vi "Data Logger.vi"(10 "logging rate (ms)":u32, 11 "YOU WANT TO LOG?":bool) -> ()   [LabVIEW 2016]
uses:
  Globale Variablen VI/AutonomousMode.vi
  Globale Variablen VI/Logging Globale Variable.vi
  Globale Variablen VI/Global Variables.vi
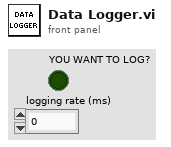
[diagram p1: front panel]
types:
  T1 = enum16{"open", "replace", "create", "open or create", "replace or create", "replace or create with confirmation"}
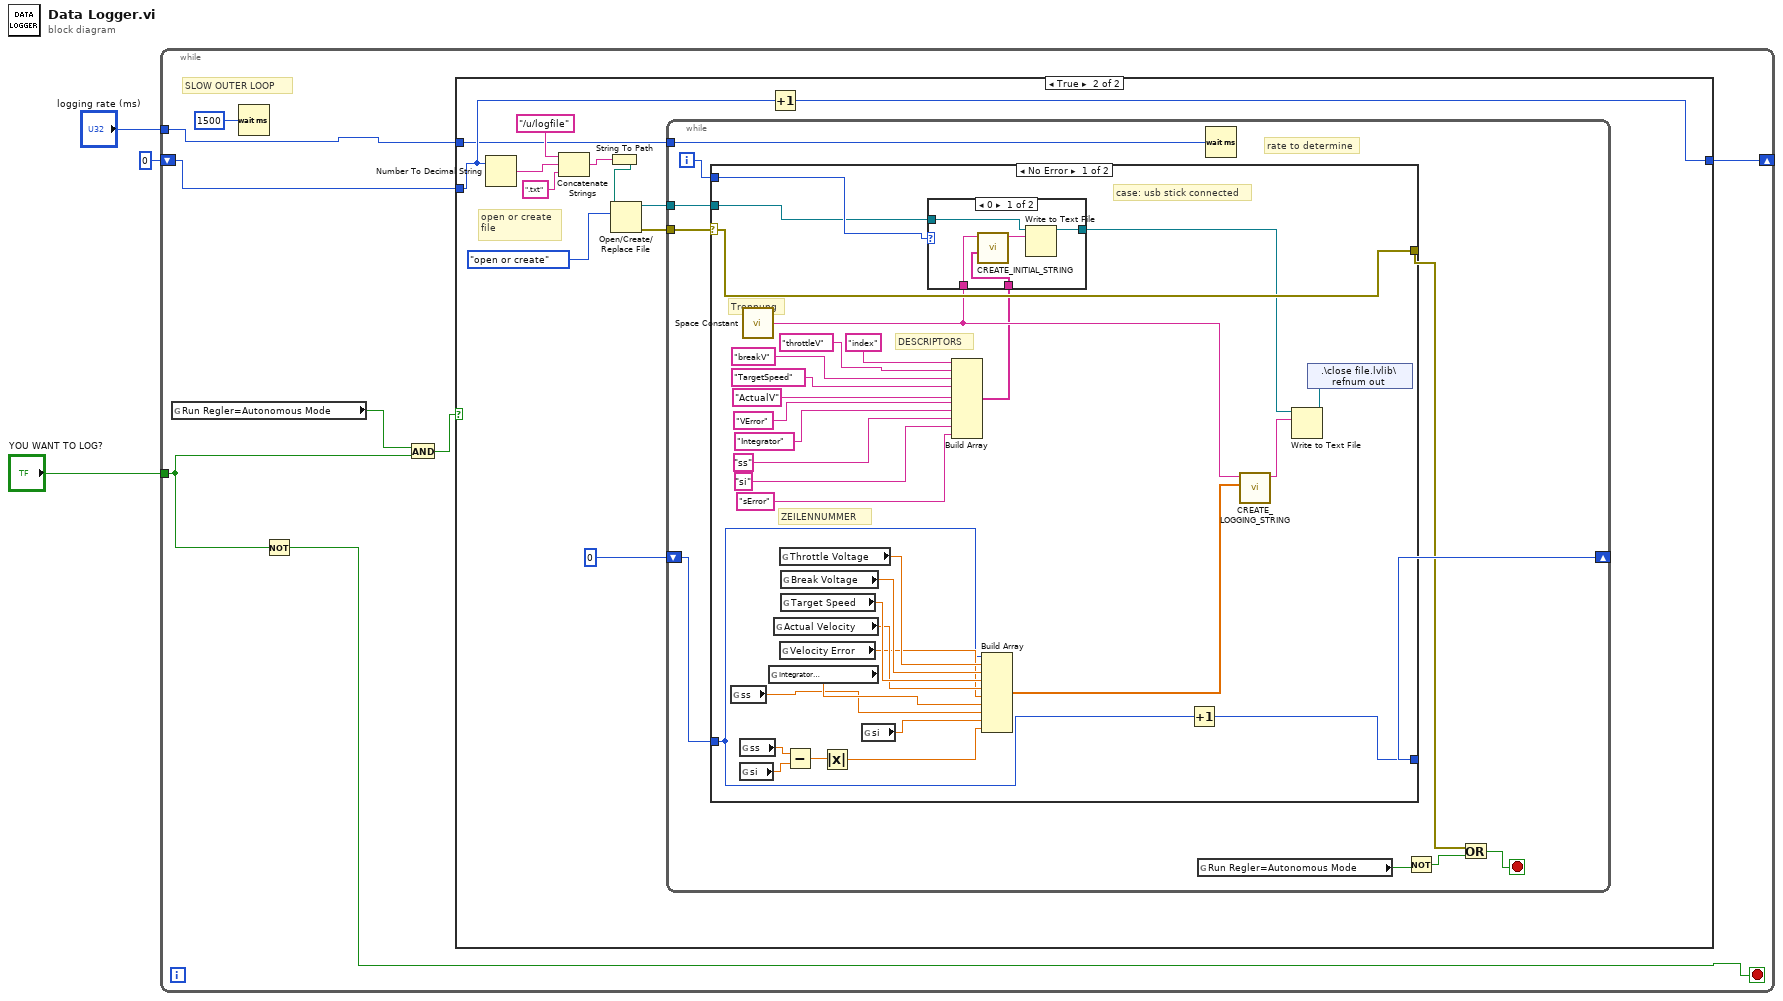
[diagram p0: block diagram]
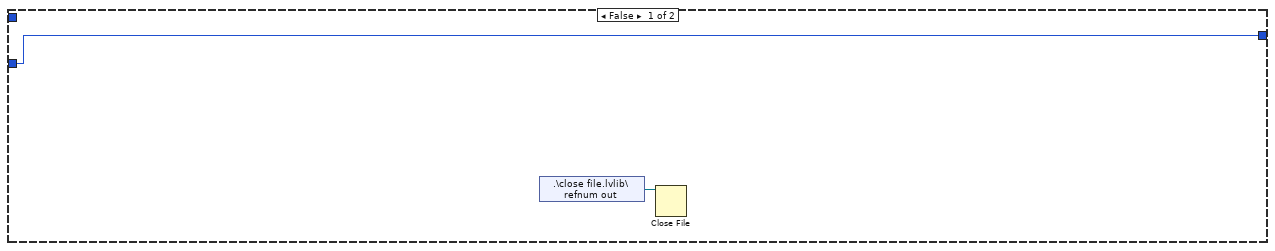
[diagram p2: hidden frame]
diagram:
  n1 = while {
    shift-right: [w10] -> _
    shift-left: i16 0 -> [w9]
    tunnel: "YOU WANT TO LOG?" -> [w6]
    tunnel: "logging rate (ms)" -> [w4]
    stop <- w5 stop-if-true
    # "SLOW OUTER LOOP"
    n2 = global read "AutonomousMode.vi" "Run Regler=Autonomous Mode"() -> (w8:bool)
    n3 = Wait (ms)(milliseconds to wait=u32 1500) -> ()  [unwired: 1 out]
    n4 = Not(x=w6) -> (.not. x?=w5:bool)
    n5 = And(x=w8, y=w6) -> (x .and. y?=w7:bool)
    n6 = case shown="True" w7 {
      tunnel: w9 -> [w13 w20]
      tunnel: [w13 w19] -> w10
      tunnel: w4 -> [_ w14]
      frame False {
        n7 = shared-variable ".\\close file.lvlib\\refnum out"() -> (w12:refnum<file>)  [unwired: 1 in, 1 out]
        n8 = Close File(refnum=w12) -> ()  [unwired: 1 in, 2 out]
      }
      frame True {
        # "open or create \nfile"
        n9 = Number To Decimal String(number=w20) -> (decimal integer string=w16:string)  [unwired: 1 in]
        n10 = Concatenate Strings("/u/logfile" ("string"), w16, ".txt") -> (w17:string)
        n11 = String To Path(string=w17) -> (path=w23:path)
        n12 = Open/Create/Replace File(file path (use dialog)=w23, operation (0:open)=T1."open or create") -> (refnum out=w21:refnum<file>, error out=w22:errorcluster)  [unwired: 4 in, 1 out]
        n13 = while {
          shift-right: [w32] -> _
          shift-left: i16 0 ("width (-)") -> [w34]
          tunnel: w22 -> [w35]
          tunnel: w21 -> [w33]
          tunnel: w14 -> [w28]
          i -> [w29]
          stop <- w31 stop-if-true
          # "rate to determine"
          n14 = case shown="No Error" w35 {
            selector: w35 -> [w59 w75]
            tunnel: [w59 w75] -> w30
            tunnel: w34 -> [w60 w76]
            tunnel: [w68 w76] -> w32
            tunnel: w33 -> [w57 _]
            tunnel: w29 -> [w58 _]
            frame No Error {
              # "Trennung"
              # "DESCRIPTORS"
              # "ZEILENNUMMER"
              # "case: usb stick connected"
              n15 = global read "Global Variables.vi" "ss"() -> (w54:dbl)
              n16 = global read "Global Variables.vi" "ss"() -> (w51:dbl)
              n17 = global read "Global Variables.vi" "si"() -> (w50:dbl)
              n18 = call <vilib>:"Space Constant.vi"() -> ("String"=w52:string)
              n19 = global read "Logging Globale Variable.vi" "Integrator\nValue"() -> (w55:dbl)
              n20 = global read "Logging Globale Variable.vi" "Actual Velocity"() -> (w64:dbl)
              n21 = global read "Logging Globale Variable.vi" "Throttle Voltage"() -> (w67:dbl)
              n22 = global read "Logging Globale Variable.vi" "Velocity Error"() -> (w63:dbl)
              n23 = global read "Logging Globale Variable.vi" "Break Voltage"() -> (w66:dbl)
              n24 = global read "Logging Globale Variable.vi" "Target Speed"() -> (w65:dbl)
              n25 = Subtract(x=w51, y=w50) -> (x-y=w49:dbl)
              n26 = Absolute Value(x=w49) -> (abs(x)=w48:dbl)
              n27 = global read "Global Variables.vi" "si"() -> (w47:dbl)
              n28 = Build Array("index", "throttleV", "breakV", "TargetSpeed", "ActualV", "VError", "Integrator", "ss", "si", "sError" ("element")) -> (w36:string[])
              n29 = case shown="0" w58 {
                tunnel: w57 -> [w73 w74]
                tunnel: [w72 w74] -> w56
                tunnel: w52 -> [w71 _]
                tunnel: w36 -> [w69 _]
                frame 0 {
                  n30 = call "CREATE_INITIAL_STRING.vi"("appended array"=w69, "String in"=w71) -> ("String out"=w70:string)  [unwired: 9 in]
                  n31 = Write to Text File(file (use dialog)=w73, text=w70) -> (refnum out=w72:refnum<file>)  [unwired: 2 in, 2 out]
                }
                frame Default {
                }
              }
              n32 = Build Array(w60, w67, w66, w65, w64, w63, w55, w54, w47, w48) -> (w62:dbl[])
              n33 = Increment(x=w60) -> (x+1=w68:i16)
              n34 = call "CREATE_LOGGING_STRING.vi"("Array"=w62, "String in"=w52) -> ("String out"=w61:string)  [unwired: 9 in]
              n35 = Write to Text File(file (use dialog)=w56, text=w61) -> (refnum out=w53:refnum<file>)  [unwired: 2 in, 2 out]
              n36 = shared-variable ".\\close file.lvlib\\refnum out"(w53) -> ()  [unwired: 1 in, 1 out]
            }
            frame Error {
              # "case: no usb stick connected"
            }
          }
          n37 = global read "AutonomousMode.vi" "Run Regler=Autonomous Mode"() -> (w27:bool)
          n38 = Wait (ms)(milliseconds to wait=w28) -> ()  [unwired: 1 out]
          n39 = Not(x=w27) -> (.not. x?=w26:bool)
          n40 = Or(x=w30, y=w26) -> (x .or. y?=w31:bool)
        }
        n41 = Increment(x=w20) -> (x+1=w19:i16)
      }
    }
  }
